vi "Try Filter Wheel.vi"() -> ()   [LabVIEW 2014]
uses:
  PAS.lvclass
panel:
  out "Numeric":i32
  out "error out":errorcluster
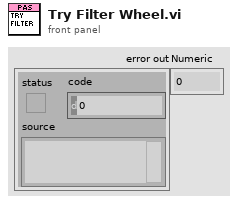
[diagram p1: front panel]
types:
  T1 = typedef "PAS.lvclass/Session Handle.ctl" = refnum<data-value>
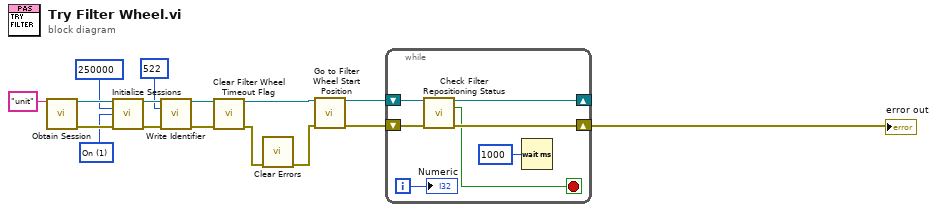
[diagram p0: block diagram]
diagram:
  w12 = u32 1 items=["Off", "On"] ("Termination")
  n1 = call "Obtain Session.vi"("Session  Name ()"="unit") -> ("Session Handle"=w16:T1, "error out"=w15:errorcluster)  [unwired: 13 in]
  n2 = call "Initialize Sessions.vi"("Session Handle in"=w16, "Baud Rate"=u32 250000, "Termination"=w12, "error in (no error)"=w15) -> ("Session Handle Out"=w11:T1, "error out"=w10:errorcluster)  [unwired: 10 in]
  n3 = call "Write Identifier.vi"("Session Handle in"=w11, "identifier"=u16 522, "error in (no error)"=w10) -> ("Session Handle out"=w5:T1, "error out"=w4:errorcluster)  [unwired: 11 in]
  n4 = call "Clear Filter Wheel Timeout Flag.vi"("Session Handle in"=w5, "error in (no error)"=w4) -> ("Session Handle out"=w1:T1, "error out"=w3:errorcluster)  [unwired: 10 in, 2 out]
  n5 = call <vilib>:"Clear Errors.vi"("error in (no error)"=w3) -> ("error out"=w2:errorcluster)  [unwired: 5 in, 1 out]
  n6 = call "Go to Filter Wheel Start Position.vi"("Session Handle in"=w1, "error in (no error)"=w2) -> ("Session Handle out"=w6:T1, "error out"=w7:errorcluster)  [unwired: 12 in]
  n7 = while {
    shift-right: [w23] -> w8
    shift-left: w7 -> [w22]
    shift-right: [w20] -> _
    shift-left: w6 -> [w21]
    i -> [w17]
    stop <- w19 stop-if-true
    n8 = call "Check Filter Repositioning Status.vi"("Session Handle in"=w21, "error in (no error)"=w22) -> ("Session Handle out"=w20:T1, "Success?"=w19:bool, "error out"=w23:errorcluster)  [unwired: 11 in]
    n9 = Wait (ms)(milliseconds to wait=u32 1000) -> ()  [unwired: 1 out]
    "Numeric" <- w17
  }
  "error out" <- w8
